vi "输入数据解析.vi"(0 "单个参数补充":dbl, 1 "从板号":dbl=1.0, 2 "主板二维码":string="BNET01", 3 "从板二维码":string="BNET01", 5 "主板引用":refnum<vi>, 7 "从板引用":refnum<vi>, 9 "主板选项":string="三级故障阀值", 11 "枚举":enum16{"主板", "从板"}(ring), 12 "快换":bool caption="快换写入") -> (4 "输出数组":dbl[][](array[numeric]), 6 "数组长度":dbl[](array[numeric]), 8 "循环次数":i32, 10 "命令":u32, 14 "名称":string[](array[string]), 15 "命令序号":u32[](array[numeric]))   [LabVIEW 2013] (continued)
                  frame Disabled {
                    n3517 = Unbundle By Name(w9112) -> ("温度过低"=w9111:dbl)
                    n3518 = call "输入分辨率计算-EV05.vi"("1字节?"=TRUE, "数值"=w9111, "偏移量"=-40.0, "分辨率"=1.0) -> ("高字节1"=w9114:dbl)  [unwired: 1 in, 6 out]
                  }
                  frame Enabled {
                  }
                }
                n3519 = Build Array(w9110) -> (w9109:i32[])
              }
              frame 4 {
                # "整组温度不均衡"
                n3520 = disable-structure shown="启用" {
                  disable-tunnel: [w9124 255 ("高字节1")] -> w9120
                  disable-tunnel: w9118 -> [w9122 _]
                  frame Disabled {
                    n3521 = Unbundle By Name(w9122) -> ("整组温度不均衡"=w9121:dbl)
                    n3522 = call "输入分辨率计算-EV05.vi"("1字节?"=TRUE, "数值"=w9121, "偏移量"=0.0, "分辨率"=1.0) -> ("高字节1"=w9124:dbl)  [unwired: 1 in, 6 out]
                  }
                  frame Enabled {
                  }
                }
                n3523 = Build Array(w9120) -> (w9119:i32[])
              }
              frame 5 {
                # "单组电压不均衡"
                n3524 = disable-structure shown="启用" {
                  disable-tunnel: [w9136 w9139] -> w9131
                  disable-tunnel: [w9134 w9139] -> w9129
                  disable-tunnel: w9128 -> [w9133 _]
                  frame Disabled {
                    n3525 = Unbundle By Name(w9133) -> ("单组电压不均衡"=w9132:dbl)
                    n3526 = call "输入分辨率计算-EV05.vi"("1字节?"=FALSE, "数值"=w9132, "偏移量"=0.0, "分辨率"=0.001) -> ("低字节"=w9134:dbl, "高字节1"=w9136:dbl)  [unwired: 1 in, 5 out]
                  }
                  frame Enabled {
                    w9139 = 255 ("高字节1")
                  }
                }
                n3527 = Build Array(w9131, w9129) -> (w9130:i32[])
              }
              frame 6 {
                # "整组电压不均衡"
                n3528 = disable-structure shown="启用" {
                  disable-tunnel: [w9148 w9151] -> w9143
                  disable-tunnel: [w9146 w9151] -> w9141
                  disable-tunnel: w9140 -> [w9145 _]
                  frame Disabled {
                    n3529 = Unbundle By Name(w9145) -> ("整组电压不均衡"=w9144:dbl)
                    n3530 = call "输入分辨率计算-EV05.vi"("1字节?"=FALSE, "数值"=w9144, "偏移量"=0.0, "分辨率"=0.001) -> ("低字节"=w9146:dbl, "高字节1"=w9148:dbl)  [unwired: 1 in, 5 out]
                  }
                  frame Enabled {
                    w9151 = 255 ("高字节1")
                  }
                }
                n3531 = Build Array(w9143, w9141) -> (w9142:i32[])
              }
              frame 7 {
                # "单体电压过高"
                n3532 = disable-structure shown="启用" {
                  disable-tunnel: [w9160 w9163] -> w9155
                  disable-tunnel: [w9158 w9163] -> w9153
                  disable-tunnel: w9152 -> [w9157 _]
                  frame Disabled {
                    n3533 = Unbundle By Name(w9157) -> ("单体电压过高"=w9156:dbl)
                    n3534 = call "输入分辨率计算-EV05.vi"("1字节?"=FALSE, "数值"=w9156, "偏移量"=0.0, "分辨率"=0.001) -> ("低字节"=w9158:dbl, "高字节1"=w9160:dbl)  [unwired: 1 in, 5 out]
                  }
                  frame Enabled {
                    w9163 = 255 ("高字节1")
                  }
                }
                n3535 = Build Array(w9155, w9153) -> (w9154:i32[])
              }
              frame 8 {
                # "单体电压过低"
                n3536 = disable-structure shown="启用" {
                  disable-tunnel: [w9172 w9175] -> w9167
                  disable-tunnel: [w9170 w9175] -> w9165
                  disable-tunnel: w9164 -> [w9169 _]
                  frame Disabled {
                    n3537 = Unbundle By Name(w9169) -> ("单体电压过低"=w9168:dbl)
                    n3538 = call "输入分辨率计算-EV05.vi"("1字节?"=FALSE, "数值"=w9168, "偏移量"=0.0, "分辨率"=0.001) -> ("低字节"=w9170:dbl, "高字节1"=w9172:dbl)  [unwired: 1 in, 5 out]
                  }
                  frame Enabled {
                    w9175 = 255 ("高字节1")
                  }
                }
                n3539 = Build Array(w9167, w9165) -> (w9166:i32[])
              }
              frame 9 {
                # "充电电流过高"
                n3540 = disable-structure shown="启用" {
                  disable-tunnel: [w9184 w9187] -> w9179
                  disable-tunnel: [w9182 w9187] -> w9177
                  disable-tunnel: w9176 -> [w9181 _]
                  frame Disabled {
                    n3541 = Unbundle By Name(w9181) -> ("充电电流过高"=w9180:dbl)
                    n3542 = call "输入分辨率计算-EV05.vi"("1字节?"=FALSE, "数值"=w9180, "偏移量"=-3000.0, "分辨率"=0.1) -> ("低字节"=w9182:dbl, "高字节1"=w9184:dbl)  [unwired: 1 in, 5 out]
                  }
                  frame Enabled {
                    w9187 = 255 ("高字节1")
                  }
                }
                n3543 = Build Array(w9179, w9177) -> (w9178:i32[])
              }
              frame 10 {
                # "放电电流过高"
                n3544 = disable-structure shown="启用" {
                  disable-tunnel: [w9196 w9199] -> w9191
                  disable-tunnel: [w9194 w9199] -> w9189
                  disable-tunnel: w9188 -> [w9193 _]
                  frame Disabled {
                    n3545 = Unbundle By Name(w9193) -> ("放电电流过高"=w9192:dbl)
                    n3546 = call "输入分辨率计算-EV05.vi"("1字节?"=FALSE, "数值"=w9192, "偏移量"=-3000.0, "分辨率"=0.1) -> ("低字节"=w9194:dbl, "高字节1"=w9196:dbl)  [unwired: 1 in, 5 out]
                  }
                  frame Enabled {
                    w9199 = 255 ("高字节1")
                  }
                }
                n3547 = Build Array(w9191, w9189) -> (w9190:i32[])
              }
              frame 11 {
                # "单组温度不均衡"
                n3548 = disable-structure shown="启用" {
                  disable-tunnel: [w9205 255 ("高字节1")] -> w9202
                  disable-tunnel: w9200 -> [w9204 _]
                  frame Enabled {
                    n3549 = Unbundle By Name(w9204) -> ("单组温度不均衡"=w9203:dbl)
                    n3550 = call "输入分辨率计算-EV05.vi"("1字节?"=TRUE, "数值"=w9203, "分辨率"=1.0) -> ("高字节1"=w9205:dbl)  [unwired: 2 in, 6 out]
                  }
                  frame Disabled {
                  }
                }
                n3551 = Build Array(w9202) -> (w9201:dbl[])
              }
              frame 12 {
                # "SOC过高"
                n3552 = Unbundle By Name(w9213) -> ("SOC过高"=w9212:dbl)
                n3553 = call "输入分辨率计算-EV05.vi"("1字节?"=FALSE, "数值"=w9212, "偏移量"=0.0, "分辨率"=0.1) -> ("低字节"=w9214:dbl, "高字节1"=w9215:dbl)  [unwired: 1 in, 5 out]
                n3554 = call "二进制解析-8.6.vi"("索引"=4, "数值"=w9215) -> ("低位子数组"=w9218:i32[])  [unwired: 3 out]
                n3555 = call "二进制解析-8.6.vi"("索引"=4, "数值"=w9214) -> ("低位子数组"=w9210:i32[], "高位子数组"=w9217:i32[])  [unwired: 2 out]
                n3556 = Insert Into Array(array=w9218, new element=w9217) -> (w9216:i32[])  [unwired: 1 in]
                n3557 = call "数值二进制转十进制-8.6.vi"("子数组"=w9216) -> ("十进制数值"=w9211:i32)  [unwired: 4 out]
                n3558 = disable-structure shown="启用" {
                  disable-tunnel: w9211 -> [w9226 _]
                  disable-tunnel: [w9226 255 ("高字节1")] -> w9209
                  disable-tunnel: w9210 -> [w9225 _]
                  disable-tunnel: [w9225 i32[] [] ("低位子数组 29")] -> _
                  frame Disabled {
                  }
                  frame Enabled {
                  }
                }
                n3559 = Build Array(w9209, w9209) -> (w9222:i32[])
              }
              frame 13 {
                # "SOC过低"
                n3560 = Unbundle By Name(w9234) -> ("SOC过低"=w9233:dbl)
                n3561 = call "输入分辨率计算-EV05.vi"("1字节?"=FALSE, "数值"=w9233, "偏移量"=0.0, "分辨率"=0.1) -> ("低字节"=w9231:dbl, "高字节1"=w9232:dbl)  [unwired: 1 in, 5 out]
                n3562 = call "二进制解析-8.6.vi"("索引"=4, "数值"=w9232) -> ("低位子数组"=w9230:i32[])  [unwired: 3 out]
                n3563 = disable-structure shown="启用" {
                  disable-tunnel: w9231 -> [w9241 _]
                  disable-tunnel: [w9241 255 ("高字节1")] -> w9229
                  disable-tunnel: w9230 -> [w9240 _]
                  disable-tunnel: [w9240 i32[] [] ("低位子数组")] -> _
                  frame Disabled {
                    (unwired) i32[] [] ("低位子数组 4")
                  }
                  frame Enabled {
                  }
                }
                n3564 = Build Array(w9229, w9229) -> (w9237:i32[])
              }
              frame 14 {
                # "内阻过大"
                n3565 = disable-structure shown="启用" {
                  disable-tunnel: w9246 -> [w9251 _]
                  disable-tunnel: [w9247 255 ("高字节1")] -> w9244
                  frame Disabled {
                    n3566 = Unbundle By Name(w9251) -> ("内阻过大"=w9250:dbl)
                    n3567 = call "输入分辨率计算-EV05.vi"("1字节?"=TRUE, "数值"=w9250, "分辨率"=0.1) -> ("高字节1"=w9247:dbl)  [unwired: 2 in, 6 out]
                  }
                  frame Enabled {
                  }
                }
                n3568 = Build Array(w9244) -> (w9245:i32[])
              }
              frame 15 {
                # "极柱温度过高"
                n3569 = disable-structure shown="启用" {
                  disable-tunnel: w9255 -> [w9261 _]
                  disable-tunnel: [w9257 255 ("高字节1")] -> w9253
                  frame Disabled {
                    n3570 = Unbundle By Name(w9261) -> ("极柱温度过高"=w9260:dbl)
                    n3571 = call "输入分辨率计算-EV05.vi"("1字节?"=TRUE, "数值"=w9260, "偏移量"=-40.0, "分辨率"=1.0) -> ("高字节1"=w9257:dbl)  [unwired: 1 in, 6 out]
                  }
                  frame Enabled {
                  }
                }
                n3572 = Build Array(w9253) -> (w9254:i32[])
              }
              frame 16 {
                # "SOH过低"
                n3573 = disable-structure shown="启用" {
                  disable-tunnel: [w9278 w9286] -> w9265
                  disable-tunnel: w9264 -> [w9275 _]
                  disable-tunnel: [w9267 w9286] -> w9263
                  frame Disabled {
                    n3574 = Unbundle By Name(w9275) -> ("SOH过低"=w9274:dbl)
                    n3575 = call "输入分辨率计算-EV05.vi"("1字节?"=FALSE, "数值"=w9274, "偏移量"=0.0, "分辨率"=0.1) -> ("低字节"=w9276:dbl, "高字节1"=w9277:dbl)  [unwired: 1 in, 5 out]
                    n3576 = call "二进制解析-8.6.vi"("索引"=4, "数值"=w9277) -> ("低位子数组"=w9280:i32[])  [unwired: 3 out]
                    n3577 = call "二进制解析-8.6.vi"("索引"=4, "数值"=w9276) -> ("低位子数组"=w9269:i32[], "高位子数组"=w9279:i32[])  [unwired: 2 out]
                    n3578 = call "二进制解析-8.6.vi"("索引"=4, "数值"=0) -> ("低位子数组"=w9270:i32[])  [unwired: 3 out]
                    n3579 = Insert Into Array(array=w9280, new element=w9279) -> (w9273:i32[])  [unwired: 1 in]
                    n3580 = Insert Into Array(array=w9269, new element=w9270) -> (w9268:i32[])  [unwired: 1 in]
                    n3581 = call "数值二进制转十进制-8.6.vi"("子数组"=w9273) -> ("十进制数值"=w9278:i32)  [unwired: 4 out]
                    n3582 = call "数值二进制转十进制-8.6.vi"("子数组"=w9268) -> ("十进制数值"=w9267:i32)  [unwired: 4 out]
                  }
                  frame Enabled {
                    w9286 = 255 ("高字节1")
                  }
                }
                n3583 = Build Array(w9265, w9263) -> (w9266:i32[])
              }
            }
            n3584 = Insert Into Array(array=w9072, new element=w9073) -> (w9071:dbl[])  [unwired: 1 in]
          }
          n3585 = Build Array(w9068) -> (w9067:dbl[][])
          n3586 = Build Array("三级故障阀值") -> (w9058:string[])
        }
        frame "内阻过大" {
          n3587 = Unbundle By Name(w9292) -> ("一级故障"=w9293:refnum<vi>)
          n3588 = property class="Clust (严格)"(reference=w9293) -> ("Value"=w9291:T4)  [unwired: 1 in, 2 out]
          n3589 = for {
            N: 17 -> [_]
            tunnel: w9291 -> [w9303]
            shift-right: [w9300] -> w9297
            shift-left: dbl[] [] -> [w9301]
            i -> [w9304]
            n3590 = case shown="13" w9304 {
              tunnel: w9303 -> [w9305 w9316 w9327 w9337 w9347 w9357 w9369 w9381 w9393 w9405 w9417 w9429 w9443 w9464 w9476 w9485 w9494]
              tunnel: [w9306 w9317 w9328 w9338 w9348 w9359 w9371 w9383 w9395 w9407 w9419 w9430 w9452 w9467 w9475 w9484 w9496] -> w9302
              frame 0, Default {
                # "总电压过高"
                n3591 = disable-structure shown="启用" {
                  disable-tunnel: [w9312 w9315] -> w9308
                  disable-tunnel: [w9311 w9315] -> w9307
                  disable-tunnel: w9305 -> [w9310 _]
                  frame Disabled {
                    n3592 = Unbundle By Name(w9310) -> ("总电压过高"=w9309:dbl)
                    n3593 = call "输入分辨率计算-EV05.vi"("1字节?"=FALSE, "数值"=w9309, "分辨率"=0.1) -> ("低字节"=w9312:dbl, "高字节1"=w9311:dbl)  [unwired: 2 in, 5 out]
                  }
                  frame Enabled {
                    w9315 = 255 ("高字节1")
                  }
                }
                n3594 = Build Array(w9307, w9308) -> (w9306:i32[])
              }
              frame 1 {
                # "总电压过低"
                n3595 = disable-structure shown="启用" {
                  disable-tunnel: [w9323 w9326] -> w9319
                  disable-tunnel: [w9322 w9326] -> w9318
                  disable-tunnel: w9316 -> [w9321 _]
                  frame Disabled {
                    n3596 = Unbundle By Name(w9321) -> ("总电压过低"=w9320:dbl)
                    n3597 = call "输入分辨率计算-EV05.vi"("1字节?"=FALSE, "数值"=w9320, "分辨率"=0.1) -> ("低字节"=w9323:dbl, "高字节1"=w9322:dbl)  [unwired: 2 in, 5 out]
                  }
                  frame Enabled {
                    w9326 = 255 ("高字节1")
                  }
                }
                n3598 = Build Array(w9318, w9319) -> (w9317:i32[])
              }
              frame 2 {
                # "温度过高"
                n3599 = disable-structure shown="启用" {
                  disable-tunnel: [w9333 255 ("高字节1")] -> w9329
                  disable-tunnel: w9327 -> [w9331 _]
                  frame Disabled {
                    n3600 = Unbundle By Name(w9331) -> ("温度过高"=w9330:dbl)
                    n3601 = call "输入分辨率计算-EV05.vi"("1字节?"=TRUE, "数值"=w9330, "偏移量"=-40.0, "分辨率"=1.0) -> ("高字节1"=w9333:dbl)  [unwired: 1 in, 6 out]
                  }
                  frame Enabled {
                  }
                }
                n3602 = Build Array(w9329) -> (w9328:i32[])
              }
              frame 3 {
                # "温度过低"
                n3603 = disable-structure shown="启用" {
                  disable-tunnel: [w9343 255 ("高字节1")] -> w9339
                  disable-tunnel: w9337 -> [w9341 _]
                  frame Disabled {
                    n3604 = Unbundle By Name(w9341) -> ("温度过低"=w9340:dbl)
                    n3605 = call "输入分辨率计算-EV05.vi"("1字节?"=TRUE, "数值"=w9340, "偏移量"=-40.0, "分辨率"=1.0) -> ("高字节1"=w9343:dbl)  [unwired: 1 in, 6 out]
                  }
                  frame Enabled {
                  }
                }
                n3606 = Build Array(w9339) -> (w9338:i32[])
              }
              frame 4 {
                # "整组温度不均衡"
                n3607 = disable-structure shown="启用" {
                  disable-tunnel: [w9353 255 ("高字节1")] -> w9349
                  disable-tunnel: w9347 -> [w9351 _]
                  frame Disabled {
                    n3608 = Unbundle By Name(w9351) -> ("整组温度不均衡"=w9350:dbl)
                    n3609 = call "输入分辨率计算-EV05.vi"("1字节?"=TRUE, "数值"=w9350, "偏移量"=0.0, "分辨率"=1.0) -> ("高字节1"=w9353:dbl)  [unwired: 1 in, 6 out]
                  }
                  frame Enabled {
                  }
                }
                n3610 = Build Array(w9349) -> (w9348:i32[])
              }
              frame 5 {
                # "单组电压不均衡"
                n3611 = disable-structure shown="启用" {
                  disable-tunnel: [w9365 w9368] -> w9360
                  disable-tunnel: [w9363 w9368] -> w9358
                  disable-tunnel: w9357 -> [w9362 _]
                  frame Disabled {
                    n3612 = Unbundle By Name(w9362) -> ("单组电压不均衡"=w9361:dbl)
                    n3613 = call "输入分辨率计算-EV05.vi"("1字节?"=FALSE, "数值"=w9361, "偏移量"=0.0, "分辨率"=0.001) -> ("低字节"=w9363:dbl, "高字节1"=w9365:dbl)  [unwired: 1 in, 5 out]
                  }
                  frame Enabled {
                    w9368 = 255 ("高字节1")
                  }
                }
                n3614 = Build Array(w9360, w9358) -> (w9359:i32[])
              }
              frame 6 {
                # "整组电压不均衡"
                n3615 = disable-structure shown="启用" {
                  disable-tunnel: [w9377 w9380] -> w9372
                  disable-tunnel: [w9375 w9380] -> w9370
                  disable-tunnel: w9369 -> [w9374 _]
                  frame Disabled {
                    n3616 = Unbundle By Name(w9374) -> ("整组电压不均衡"=w9373:dbl)
                    n3617 = call "输入分辨率计算-EV05.vi"("1字节?"=FALSE, "数值"=w9373, "偏移量"=0.0, "分辨率"=0.001) -> ("低字节"=w9375:dbl, "高字节1"=w9377:dbl)  [unwired: 1 in, 5 out]
                  }
                  frame Enabled {
                    w9380 = 255 ("高字节1")
                  }
                }
                n3618 = Build Array(w9372, w9370) -> (w9371:i32[])
              }
              frame 7 {
                # "单体电压过高"
                n3619 = disable-structure shown="启用" {
                  disable-tunnel: [w9389 w9392] -> w9384
                  disable-tunnel: [w9387 w9392] -> w9382
                  disable-tunnel: w9381 -> [w9386 _]
                  frame Disabled {
                    n3620 = Unbundle By Name(w9386) -> ("单体电压过高"=w9385:dbl)
                    n3621 = call "输入分辨率计算-EV05.vi"("1字节?"=FALSE, "数值"=w9385, "偏移量"=0.0, "分辨率"=0.001) -> ("低字节"=w9387:dbl, "高字节1"=w9389:dbl)  [unwired: 1 in, 5 out]
                  }
                  frame Enabled {
                    w9392 = 255 ("高字节1")
                  }
                }
                n3622 = Build Array(w9384, w9382) -> (w9383:i32[])
              }
              frame 8 {
                # "单体电压过低"
                n3623 = disable-structure shown="启用" {
                  disable-tunnel: [w9401 w9404] -> w9396
                  disable-tunnel: [w9399 w9404] -> w9394
                  disable-tunnel: w9393 -> [w9398 _]
                  frame Disabled {
                    n3624 = Unbundle By Name(w9398) -> ("单体电压过低"=w9397:dbl)
                    n3625 = call "输入分辨率计算-EV05.vi"("1字节?"=FALSE, "数值"=w9397, "偏移量"=0.0, "分辨率"=0.001) -> ("低字节"=w9399:dbl, "高字节1"=w9401:dbl)  [unwired: 1 in, 5 out]
                  }
                  frame Enabled {
                    w9404 = 255 ("高字节1")
                  }
                }
                n3626 = Build Array(w9396, w9394) -> (w9395:i32[])
              }
              frame 9 {
                # "充电电流过高"
                n3627 = disable-structure shown="启用" {
                  disable-tunnel: [w9413 w9416] -> w9408
                  disable-tunnel: [w9411 w9416] -> w9406
                  disable-tunnel: w9405 -> [w9410 _]
                  frame Disabled {
                    n3628 = Unbundle By Name(w9410) -> ("充电电流过高"=w9409:dbl)
                    n3629 = call "输入分辨率计算-EV05.vi"("1字节?"=FALSE, "数值"=w9409, "偏移量"=-3000.0, "分辨率"=0.1) -> ("低字节"=w9411:dbl, "高字节1"=w9413:dbl)  [unwired: 1 in, 5 out]
                  }
                  frame Enabled {
                    w9416 = 255 ("高字节1")
                  }
                }
                n3630 = Build Array(w9408, w9406) -> (w9407:i32[])
              }
              frame 10 {
                # "放电电流过高"
                n3631 = disable-structure shown="启用" {
                  disable-tunnel: [w9425 w9428] -> w9420
                  disable-tunnel: [w9423 w9428] -> w9418
                  disable-tunnel: w9417 -> [w9422 _]
                  frame Disabled {
                    n3632 = Unbundle By Name(w9422) -> ("放电电流过高"=w9421:dbl)
                    n3633 = call "输入分辨率计算-EV05.vi"("1字节?"=FALSE, "数值"=w9421, "偏移量"=-3000.0, "分辨率"=0.1) -> ("低字节"=w9423:dbl, "高字节1"=w9425:dbl)  [unwired: 1 in, 5 out]
                  }
                  frame Enabled {
                    w9428 = 255 ("高字节1")
                  }
                }
                n3634 = Build Array(w9420, w9418) -> (w9419:i32[])
              }
              frame 11 {
                # "单组温度不均衡"
                n3635 = disable-structure shown="启用" {
                  disable-tunnel: [w9435 255 ("高字节1")] -> w9431
                  disable-tunnel: w9429 -> [w9433 _]
                  frame Disabled {
                    n3636 = Unbundle By Name(w9433) -> ("单组温度不均衡"=w9432:dbl)
                    n3637 = call "输入分辨率计算-EV05.vi"("1字节?"=TRUE, "数值"=w9432, "偏移量"=0.0, "分辨率"=1.0) -> ("高字节1"=w9435:dbl)  [unwired: 1 in, 6 out]
                  }
                  frame Enabled {
                  }
                }
                n3638 = Build Array(w9431) -> (w9430:i32[])
              }
              frame 12 {
                # "SOC过高"
                n3639 = Unbundle By Name(w9443) -> ("SOC过高"=w9442:dbl)
                n3640 = call "输入分辨率计算-EV05.vi"("1字节?"=FALSE, "数值"=w9442, "偏移量"=0.0, "分辨率"=0.1) -> ("低字节"=w9444:dbl, "高字节1"=w9445:dbl)  [unwired: 1 in, 5 out]
                n3641 = call "二进制解析-8.6.vi"("索引"=4, "数值"=w9445) -> ("低位子数组"=w9448:i32[])  [unwired: 3 out]
                n3642 = call "二进制解析-8.6.vi"("索引"=4, "数值"=w9444) -> ("低位子数组"=w9440:i32[], "高位子数组"=w9447:i32[])  [unwired: 2 out]
                n3643 = Insert Into Array(array=w9448, new element=w9447) -> (w9446:i32[])  [unwired: 1 in]
                n3644 = call "数值二进制转十进制-8.6.vi"("子数组"=w9446) -> ("十进制数值"=w9441:i32)  [unwired: 4 out]
                n3645 = disable-structure shown="启用" {
                  disable-tunnel: w9441 -> [w9456 _]
                  disable-tunnel: [w9456 255 ("高字节1")] -> w9439
                  disable-tunnel: w9440 -> [w9455 _]
                  disable-tunnel: [w9455 i32[] [] ("低位子数组 29")] -> _
                  frame Disabled {
                  }
                  frame Enabled {
                  }
                }
                n3646 = Build Array(w9439, w9439) -> (w9452:i32[])
              }
              frame 13 {
                # "SOC过低"
                n3647 = Unbundle By Name(w9464) -> ("SOC过低"=w9463:dbl)
                n3648 = call "输入分辨率计算-EV05.vi"("1字节?"=FALSE, "数值"=w9463, "偏移量"=0.0, "分辨率"=0.1) -> ("低字节"=w9461:dbl, "高字节1"=w9462:dbl)  [unwired: 1 in, 5 out]
                n3649 = call "二进制解析-8.6.vi"("索引"=4, "数值"=w9462) -> ("低位子数组"=w9460:i32[])  [unwired: 3 out]
                n3650 = disable-structure shown="启用" {
                  disable-tunnel: w9461 -> [w9471 _]
                  disable-tunnel: [w9471 255 ("高字节1")] -> w9459
                  disable-tunnel: w9460 -> [w9470 _]
                  disable-tunnel: [w9470 i32[] [] ("低位子数组")] -> _
                  frame Disabled {
                    (unwired) i32[] [] ("低位子数组 4")
                  }
                  frame Enabled {
                  }
                }
                n3651 = Build Array(w9459, w9459) -> (w9467:i32[])
              }
              frame 14 {
                # "内阻过大"
                n3652 = disable-structure shown="启用" {
                  disable-tunnel: w9476 -> [w9481 _]
                  disable-tunnel: [w9477 255 ("高字节1")] -> w9474
                  frame Enabled {
                    n3653 = Unbundle By Name(w9481) -> ("内阻过大"=w9480:dbl)
                    n3654 = call "输入分辨率计算-EV05.vi"("1字节?"=TRUE, "数值"=w9480, "分辨率"=0.1) -> ("高字节1"=w9477:dbl)  [unwired: 2 in, 6 out]
                  }
                  frame Disabled {
                  }
                }
                n3655 = Build Array(w9474) -> (w9475:dbl[])
              }
              frame 15 {
                # "极柱温度过高"
                n3656 = disable-structure shown="启用" {
                  disable-tunnel: w9485 -> [w9491 _]
                  disable-tunnel: [w9487 255 ("高字节1")] -> w9483
                  frame Disabled {
                    n3657 = Unbundle By Name(w9491) -> ("极柱温度过高"=w9490:dbl)
                    n3658 = call "输入分辨率计算-EV05.vi"("1字节?"=TRUE, "数值"=w9490, "偏移量"=-40.0, "分辨率"=1.0) -> ("高字节1"=w9487:dbl)  [unwired: 1 in, 6 out]
                  }
                  frame Enabled {
                  }
                }
                n3659 = Build Array(w9483) -> (w9484:i32[])
              }
              frame 16 {
                # "SOH过低"
                n3660 = disable-structure shown="启用" {
                  disable-tunnel: [w9508 w9516] -> w9495
                  disable-tunnel: w9494 -> [w9505 _]
                  disable-tunnel: [w9497 w9516] -> w9493
                  frame Disabled {
                    n3661 = Unbundle By Name(w9505) -> ("SOH过低"=w9504:dbl)
                    n3662 = call "输入分辨率计算-EV05.vi"("1字节?"=FALSE, "数值"=w9504, "偏移量"=0.0, "分辨率"=0.1) -> ("低字节"=w9506:dbl, "高字节1"=w9507:dbl)  [unwired: 1 in, 5 out]
                    n3663 = call "二进制解析-8.6.vi"("索引"=4, "数值"=w9507) -> ("低位子数组"=w9510:i32[])  [unwired: 3 out]
                    n3664 = call "二进制解析-8.6.vi"("索引"=4, "数值"=w9506) -> ("低位子数组"=w9499:i32[], "高位子数组"=w9509:i32[])  [unwired: 2 out]
                    n3665 = call "二进制解析-8.6.vi"("索引"=4, "数值"=0) -> ("低位子数组"=w9500:i32[])  [unwired: 3 out]
                    n3666 = Insert Into Array(array=w9510, new element=w9509) -> (w9503:i32[])  [unwired: 1 in]
                    n3667 = Insert Into Array(array=w9499, new element=w9500) -> (w9498:i32[])  [unwired: 1 in]
                    n3668 = call "数值二进制转十进制-8.6.vi"("子数组"=w9503) -> ("十进制数值"=w9508:i32)  [unwired: 4 out]
                    n3669 = call "数值二进制转十进制-8.6.vi"("子数组"=w9498) -> ("十进制数值"=w9497:i32)  [unwired: 4 out]
                  }
                  frame Enabled {
                    w9516 = 255 ("高字节1")
                  }
                }
                n3670 = Build Array(w9495, w9493) -> (w9496:i32[])
              }
            }
            n3671 = Insert Into Array(array=w9301, new element=w9302) -> (w9300:dbl[])  [unwired: 1 in]
          }
          n3672 = Build Array(w9297) -> (w9296:dbl[][])
          n3673 = Build Array("一级故障阀值") -> (w9287:string[])
        }
        frame "内阻过大(2)" {
          n3674 = Unbundle By Name(w9522) -> ("一级故障 2"=w9523:refnum<vi>)
          n3675 = property class="Clust (严格)"(reference=w9523) -> ("Value"=w9521:T4)  [unwired: 1 in, 2 out]
          n3676 = for {
            N: 17 -> [_]
            tunnel: w9521 -> [w9533]
            shift-right: [w9530] -> w9527
            shift-left: dbl[] [] -> [w9531]
            i -> [w9534]
            n3677 = case shown="13" w9534 {
              tunnel: w9533 -> [w9535 w9546 w9557 w9567 w9577 w9587 w9599 w9611 w9623 w9635 w9647 w9659 w9673 w9694 w9706 w9715 w9724]
              tunnel: [w9536 w9547 w9558 w9568 w9578 w9589 w9601 w9613 w9625 w9637 w9649 w9660 w9682 w9697 w9705 w9714 w9726] -> w9532
              frame 0, Default {
                # "总电压过高"
                n3678 = disable-structure shown="启用" {
                  disable-tunnel: [w9542 w9545] -> w9538
                  disable-tunnel: [w9541 w9545] -> w9537
                  disable-tunnel: w9535 -> [w9540 _]
                  frame Disabled {
                    n3679 = Unbundle By Name(w9540) -> ("总电压过高"=w9539:dbl)
                    n3680 = call "输入分辨率计算-EV05.vi"("1字节?"=FALSE, "数值"=w9539, "分辨率"=0.1) -> ("低字节"=w9542:dbl, "高字节1"=w9541:dbl)  [unwired: 2 in, 5 out]
                  }
                  frame Enabled {
                    w9545 = 255 ("高字节1")
                  }
                }
                n3681 = Build Array(w9537, w9538) -> (w9536:i32[])
              }
              frame 1 {
                # "总电压过低"
                n3682 = disable-structure shown="启用" {
                  disable-tunnel: [w9553 w9556] -> w9549
                  disable-tunnel: [w9552 w9556] -> w9548
                  disable-tunnel: w9546 -> [w9551 _]
                  frame Disabled {
                    n3683 = Unbundle By Name(w9551) -> ("总电压过低"=w9550:dbl)
                    n3684 = call "输入分辨率计算-EV05.vi"("1字节?"=FALSE, "数值"=w9550, "分辨率"=0.1) -> ("低字节"=w9553:dbl, "高字节1"=w9552:dbl)  [unwired: 2 in, 5 out]
                  }
                  frame Enabled {
                    w9556 = 255 ("高字节1")
                  }
                }
                n3685 = Build Array(w9548, w9549) -> (w9547:i32[])
              }
              frame 2 {
                # "温度过高"
                n3686 = disable-structure shown="启用" {
                  disable-tunnel: [w9563 255 ("高字节1")] -> w9559
                  disable-tunnel: w9557 -> [w9561 _]
                  frame Disabled {
                    n3687 = Unbundle By Name(w9561) -> ("温度过高"=w9560:dbl)
                    n3688 = call "输入分辨率计算-EV05.vi"("1字节?"=TRUE, "数值"=w9560, "偏移量"=-40.0, "分辨率"=1.0) -> ("高字节1"=w9563:dbl)  [unwired: 1 in, 6 out]
                  }
                  frame Enabled {
                  }
                }
                n3689 = Build Array(w9559) -> (w9558:i32[])
              }
              frame 3 {
                # "温度过低"
                n3690 = disable-structure shown="启用" {
                  disable-tunnel: [w9573 255 ("高字节1")] -> w9569
                  disable-tunnel: w9567 -> [w9571 _]
                  frame Disabled {
                    n3691 = Unbundle By Name(w9571) -> ("温度过低"=w9570:dbl)
                    n3692 = call "输入分辨率计算-EV05.vi"("1字节?"=TRUE, "数值"=w9570, "偏移量"=-40.0, "分辨率"=1.0) -> ("高字节1"=w9573:dbl)  [unwired: 1 in, 6 out]
                  }
                  frame Enabled {
                  }
                }
                n3693 = Build Array(w9569) -> (w9568:i32[])
              }
              frame 4 {
                # "整组温度不均衡"
                n3694 = disable-structure shown="启用" {
                  disable-tunnel: [w9583 255 ("高字节1")] -> w9579
                  disable-tunnel: w9577 -> [w9581 _]
                  frame Disabled {
                    n3695 = Unbundle By Name(w9581) -> ("整组温度不均衡"=w9580:dbl)
                    n3696 = call "输入分辨率计算-EV05.vi"("1字节?"=TRUE, "数值"=w9580, "偏移量"=0.0, "分辨率"=1.0) -> ("高字节1"=w9583:dbl)  [unwired: 1 in, 6 out]
                  }
                  frame Enabled {
                  }
                }
                n3697 = Build Array(w9579) -> (w9578:i32[])
              }
              frame 5 {
                # "单组电压不均衡"
                n3698 = disable-structure shown="启用" {
                  disable-tunnel: [w9595 w9598] -> w9590
                  disable-tunnel: [w9593 w9598] -> w9588
                  disable-tunnel: w9587 -> [w9592 _]
                  frame Disabled {
                    n3699 = Unbundle By Name(w9592) -> ("单组电压不均衡"=w9591:dbl)
                    n3700 = call "输入分辨率计算-EV05.vi"("1字节?"=FALSE, "数值"=w9591, "偏移量"=0.0, "分辨率"=0.001) -> ("低字节"=w9593:dbl, "高字节1"=w9595:dbl)  [unwired: 1 in, 5 out]
                  }
                  frame Enabled {
                    w9598 = 255 ("高字节1")
                  }
                }
                n3701 = Build Array(w9590, w9588) -> (w9589:i32[])
              }
              frame 6 {
                # "整组电压不均衡"
                n3702 = disable-structure shown="启用" {
                  disable-tunnel: [w9607 w9610] -> w9602
                  disable-tunnel: [w9605 w9610] -> w9600
                  disable-tunnel: w9599 -> [w9604 _]
                  frame Disabled {
                    n3703 = Unbundle By Name(w9604) -> ("整组电压不均衡"=w9603:dbl)
                    n3704 = call "输入分辨率计算-EV05.vi"("1字节?"=FALSE, "数值"=w9603, "偏移量"=0.0, "分辨率"=0.001) -> ("低字节"=w9605:dbl, "高字节1"=w9607:dbl)  [unwired: 1 in, 5 out]
                  }
                  frame Enabled {
                    w9610 = 255 ("高字节1")
                  }
                }
                n3705 = Build Array(w9602, w9600) -> (w9601:i32[])
              }
              frame 7 {
                # "单体电压过高"
                n3706 = disable-structure shown="启用" {
                  disable-tunnel: [w9619 w9622] -> w9614
                  disable-tunnel: [w9617 w9622] -> w9612
                  disable-tunnel: w9611 -> [w9616 _]
                  frame Disabled {
                    n3707 = Unbundle By Name(w9616) -> ("单体电压过高"=w9615:dbl)
                    n3708 = call "输入分辨率计算-EV05.vi"("1字节?"=FALSE, "数值"=w9615, "偏移量"=0.0, "分辨率"=0.001) -> ("低字节"=w9617:dbl, "高字节1"=w9619:dbl)  [unwired: 1 in, 5 out]
                  }
                  frame Enabled {
                    w9622 = 255 ("高字节1")
                  }
                }
                n3709 = Build Array(w9614, w9612) -> (w9613:i32[])
              }
              frame 8 {
                # "单体电压过低"
                n3710 = disable-structure shown="启用" {
                  disable-tunnel: [w9631 w9634] -> w9626
                  disable-tunnel: [w9629 w9634] -> w9624
                  disable-tunnel: w9623 -> [w9628 _]
                  frame Disabled {
                    n3711 = Unbundle By Name(w9628) -> ("单体电压过低"=w9627:dbl)
                    n3712 = call "输入分辨率计算-EV05.vi"("1字节?"=FALSE, "数值"=w9627, "偏移量"=0.0, "分辨率"=0.001) -> ("低字节"=w9629:dbl, "高字节1"=w9631:dbl)  [unwired: 1 in, 5 out]
                  }
                  frame Enabled {
                    w9634 = 255 ("高字节1")
                  }
                }
                n3713 = Build Array(w9626, w9624) -> (w9625:i32[])
              }
              frame 9 {
                # "充电电流过高"
                n3714 = disable-structure shown="启用" {
                  disable-tunnel: [w9643 w9646] -> w9638
                  disable-tunnel: [w9641 w9646] -> w9636
                  disable-tunnel: w9635 -> [w9640 _]
                  frame Disabled {
                    n3715 = Unbundle By Name(w9640) -> ("充电电流过高"=w9639:dbl)
                    n3716 = call "输入分辨率计算-EV05.vi"("1字节?"=FALSE, "数值"=w9639, "偏移量"=-3000.0, "分辨率"=0.1) -> ("低字节"=w9641:dbl, "高字节1"=w9643:dbl)  [unwired: 1 in, 5 out]
                  }
                  frame Enabled {
                    w9646 = 255 ("高字节1")
                  }
                }
                n3717 = Build Array(w9638, w9636) -> (w9637:i32[])
              }
              frame 10 {
                # "放电电流过高"
                n3718 = disable-structure shown="启用" {
                  disable-tunnel: [w9655 w9658] -> w9650
                  disable-tunnel: [w9653 w9658] -> w9648
                  disable-tunnel: w9647 -> [w9652 _]
                  frame Disabled {
                    n3719 = Unbundle By Name(w9652) -> ("放电电流过高"=w9651:dbl)
                    n3720 = call "输入分辨率计算-EV05.vi"("1字节?"=FALSE, "数值"=w9651, "偏移量"=-3000.0, "分辨率"=0.1) -> ("低字节"=w9653:dbl, "高字节1"=w9655:dbl)  [unwired: 1 in, 5 out]
                  }
                  frame Enabled {
                    w9658 = 255 ("高字节1")
                  }
                }
                n3721 = Build Array(w9650, w9648) -> (w9649:i32[])
              }
              frame 11 {
                # "单组温度不均衡"
                n3722 = disable-structure shown="启用" {
                  disable-tunnel: [w9665 255 ("高字节1")] -> w9661
                  disable-tunnel: w9659 -> [w9663 _]
                  frame Disabled {
                    n3723 = Unbundle By Name(w9663) -> ("单组温度不均衡"=w9662:dbl)
                    n3724 = call "输入分辨率计算-EV05.vi"("1字节?"=TRUE, "数值"=w9662, "偏移量"=0.0, "分辨率"=1.0) -> ("高字节1"=w9665:dbl)  [unwired: 1 in, 6 out]
                  }
                  frame Enabled {
                  }
                }
                n3725 = Build Array(w9661) -> (w9660:i32[])
              }
              frame 12 {
                # "SOC过高"
                n3726 = Unbundle By Name(w9673) -> ("SOC过高"=w9672:dbl)
                n3727 = call "输入分辨率计算-EV05.vi"("1字节?"=FALSE, "数值"=w9672, "偏移量"=0.0, "分辨率"=0.1) -> ("低字节"=w9674:dbl, "高字节1"=w9675:dbl)  [unwired: 1 in, 5 out]
                n3728 = call "二进制解析-8.6.vi"("索引"=4, "数值"=w9675) -> ("低位子数组"=w9678:i32[])  [unwired: 3 out]
                n3729 = call "二进制解析-8.6.vi"("索引"=4, "数值"=w9674) -> ("低位子数组"=w9670:i32[], "高位子数组"=w9677:i32[])  [unwired: 2 out]
                n3730 = Insert Into Array(array=w9678, new element=w9677) -> (w9676:i32[])  [unwired: 1 in]
                n3731 = call "数值二进制转十进制-8.6.vi"("子数组"=w9676) -> ("十进制数值"=w9671:i32)  [unwired: 4 out]
                n3732 = disable-structure shown="启用" {
                  disable-tunnel: w9671 -> [w9686 _]
                  disable-tunnel: [w9686 255 ("高字节1")] -> w9669
                  disable-tunnel: w9670 -> [w9685 _]
                  disable-tunnel: [w9685 i32[] [] ("低位子数组 29")] -> _
                  frame Disabled {
                  }
                  frame Enabled {
                  }
                }
                n3733 = Build Array(w9669, w9669) -> (w9682:i32[])
              }
              frame 13 {
                # "SOC过低"
                n3734 = Unbundle By Name(w9694) -> ("SOC过低"=w9693:dbl)
                n3735 = call "输入分辨率计算-EV05.vi"("1字节?"=FALSE, "数值"=w9693, "偏移量"=0.0, "分辨率"=0.1) -> ("低字节"=w9691:dbl, "高字节1"=w9692:dbl)  [unwired: 1 in, 5 out]
                n3736 = call "二进制解析-8.6.vi"("索引"=4, "数值"=w9692) -> ("低位子数组"=w9690:i32[])  [unwired: 3 out]
                n3737 = disable-structure shown="启用" {
                  disable-tunnel: w9691 -> [w9701 _]
                  disable-tunnel: [w9701 255 ("高字节1")] -> w9689
                  disable-tunnel: w9690 -> [w9700 _]
                  disable-tunnel: [w9700 i32[] [] ("低位子数组")] -> _
                  frame Disabled {
                    (unwired) i32[] [] ("低位子数组 4")
                  }
                  frame Enabled {
                  }
                }
                n3738 = Build Array(w9689, w9689) -> (w9697:i32[])
              }
              frame 14 {
                # "内阻过大"
                n3739 = disable-structure shown="启用" {
                  disable-tunnel: w9706 -> [w9711 _]
                  disable-tunnel: [w9707 255 ("高字节1")] -> w9704
                  frame Enabled {
                    n3740 = Unbundle By Name(w9711) -> ("内阻过大"=w9710:dbl)
                    n3741 = call "输入分辨率计算-EV05.vi"("1字节?"=TRUE, "数值"=w9710, "分辨率"=0.1) -> ("高字节1"=w9707:dbl)  [unwired: 2 in, 6 out]
                  }
                  frame Disabled {
                  }
                }
                n3742 = Build Array(w9704) -> (w9705:dbl[])
              }
              frame 15 {
                # "极柱温度过高"
                n3743 = disable-structure shown="启用" {
                  disable-tunnel: w9715 -> [w9721 _]
                  disable-tunnel: [w9717 255 ("高字节1")] -> w9713
                  frame Disabled {
                    n3744 = Unbundle By Name(w9721) -> ("极柱温度过高"=w9720:dbl)
                    n3745 = call "输入分辨率计算-EV05.vi"("1字节?"=TRUE, "数值"=w9720, "偏移量"=-40.0, "分辨率"=1.0) -> ("高字节1"=w9717:dbl)  [unwired: 1 in, 6 out]
                  }
                  frame Enabled {
                  }
                }
                n3746 = Build Array(w9713) -> (w9714:i32[])
              }
              frame 16 {
                # "SOH过低"
                n3747 = disable-structure shown="启用" {
                  disable-tunnel: [w9738 w9746] -> w9725
                  disable-tunnel: w9724 -> [w9735 _]
                  disable-tunnel: [w9727 w9746] -> w9723
                  frame Disabled {
                    n3748 = Unbundle By Name(w9735) -> ("SOH过低"=w9734:dbl)
                    n3749 = call "输入分辨率计算-EV05.vi"("1字节?"=FALSE, "数值"=w9734, "偏移量"=0.0, "分辨率"=0.1) -> ("低字节"=w9736:dbl, "高字节1"=w9737:dbl)  [unwired: 1 in, 5 out]
                    n3750 = call "二进制解析-8.6.vi"("索引"=4, "数值"=w9737) -> ("低位子数组"=w9740:i32[])  [unwired: 3 out]
                    n3751 = call "二进制解析-8.6.vi"("索引"=4, "数值"=w9736) -> ("低位子数组"=w9729:i32[], "高位子数组"=w9739:i32[])  [unwired: 2 out]
                    n3752 = call "二进制解析-8.6.vi"("索引"=4, "数值"=0) -> ("低位子数组"=w9730:i32[])  [unwired: 3 out]
                    n3753 = Insert Into Array(array=w9740, new element=w9739) -> (w9733:i32[])  [unwired: 1 in]
                    n3754 = Insert Into Array(array=w9729, new element=w9730) -> (w9728:i32[])  [unwired: 1 in]
                    n3755 = call "数值二进制转十进制-8.6.vi"("子数组"=w9733) -> ("十进制数值"=w9738:i32)  [unwired: 4 out]
                    n3756 = call "数值二进制转十进制-8.6.vi"("子数组"=w9728) -> ("十进制数值"=w9727:i32)  [unwired: 4 out]
                  }
                  frame Enabled {
                    w9746 = 255 ("高字节1")
                  }
                }
                n3757 = Build Array(w9725, w9723) -> (w9726:i32[])
              }
            }
            n3758 = Insert Into Array(array=w9531, new element=w9532) -> (w9530:dbl[])  [unwired: 1 in]
          }
          n3759 = Build Array(w9527) -> (w9526:dbl[][])
          n3760 = Build Array("二级故障阀值") -> (w9517:string[])
        }
        frame "内阻过大(3)" {
          n3761 = Unbundle By Name(w9752) -> ("一级故障 3"=w9753:refnum<vi>)
          n3762 = property class="Clust (严格)"(reference=w9753) -> ("Value"=w9751:T4)  [unwired: 1 in, 2 out]
          n3763 = for {
            N: 17 -> [_]
            tunnel: w9751 -> [w9763]
            shift-right: [w9760] -> w9757
            shift-left: dbl[] [] -> [w9761]
            i -> [w9764]
            n3764 = case shown="13" w9764 {
              tunnel: w9763 -> [w9765 w9776 w9787 w9797 w9807 w9817 w9829 w9841 w9853 w9865 w9877 w9889 w9903 w9924 w9936 w9945 w9954]
              tunnel: [w9766 w9777 w9788 w9798 w9808 w9819 w9831 w9843 w9855 w9867 w9879 w9890 w9912 w9927 w9935 w9944 w9956] -> w9762
              frame 0, Default {
                # "总电压过高"
                n3765 = disable-structure shown="启用" {
                  disable-tunnel: [w9772 w9775] -> w9768
                  disable-tunnel: [w9771 w9775] -> w9767
                  disable-tunnel: w9765 -> [w9770 _]
                  frame Disabled {
                    n3766 = Unbundle By Name(w9770) -> ("总电压过高"=w9769:dbl)
                    n3767 = call "输入分辨率计算-EV05.vi"("1字节?"=FALSE, "数值"=w9769, "分辨率"=0.1) -> ("低字节"=w9772:dbl, "高字节1"=w9771:dbl)  [unwired: 2 in, 5 out]
                  }
                  frame Enabled {
                    w9775 = 255 ("高字节1")
                  }
                }
                n3768 = Build Array(w9767, w9768) -> (w9766:i32[])
              }
              frame 1 {
                # "总电压过低"
                n3769 = disable-structure shown="启用" {
                  disable-tunnel: [w9783 w9786] -> w9779
                  disable-tunnel: [w9782 w9786] -> w9778
                  disable-tunnel: w9776 -> [w9781 _]
                  frame Disabled {
                    n3770 = Unbundle By Name(w9781) -> ("总电压过低"=w9780:dbl)
                    n3771 = call "输入分辨率计算-EV05.vi"("1字节?"=FALSE, "数值"=w9780, "分辨率"=0.1) -> ("低字节"=w9783:dbl, "高字节1"=w9782:dbl)  [unwired: 2 in, 5 out]
                  }
                  frame Enabled {
                    w9786 = 255 ("高字节1")
                  }
                }
                n3772 = Build Array(w9778, w9779) -> (w9777:i32[])
              }
              frame 2 {
                # "温度过高"
                n3773 = disable-structure shown="启用" {
                  disable-tunnel: [w9793 255 ("高字节1")] -> w9789
                  disable-tunnel: w9787 -> [w9791 _]
                  frame Disabled {
                    n3774 = Unbundle By Name(w9791) -> ("温度过高"=w9790:dbl)
                    n3775 = call "输入分辨率计算-EV05.vi"("1字节?"=TRUE, "数值"=w9790, "偏移量"=-40.0, "分辨率"=1.0) -> ("高字节1"=w9793:dbl)  [unwired: 1 in, 6 out]
                  }
                  frame Enabled {
                  }
                }
                n3776 = Build Array(w9789) -> (w9788:i32[])
              }
              frame 3 {
                # "温度过低"
                n3777 = disable-structure shown="启用" {
                  disable-tunnel: [w9803 255 ("高字节1")] -> w9799
                  disable-tunnel: w9797 -> [w9801 _]
                  frame Disabled {
                    n3778 = Unbundle By Name(w9801) -> ("温度过低"=w9800:dbl)
                    n3779 = call "输入分辨率计算-EV05.vi"("1字节?"=TRUE, "数值"=w9800, "偏移量"=-40.0, "分辨率"=1.0) -> ("高字节1"=w9803:dbl)  [unwired: 1 in, 6 out]
                  }
                  frame Enabled {
                  }
                }
                n3780 = Build Array(w9799) -> (w9798:i32[])
              }
              frame 4 {
                # "整组温度不均衡"
                n3781 = disable-structure shown="启用" {
                  disable-tunnel: [w9813 255 ("高字节1")] -> w9809
                  disable-tunnel: w9807 -> [w9811 _]
                  frame Disabled {
                    n3782 = Unbundle By Name(w9811) -> ("整组温度不均衡"=w9810:dbl)
                    n3783 = call "输入分辨率计算-EV05.vi"("1字节?"=TRUE, "数值"=w9810, "偏移量"=0.0, "分辨率"=1.0) -> ("高字节1"=w9813:dbl)  [unwired: 1 in, 6 out]
                  }
                  frame Enabled {
                  }
                }
                n3784 = Build Array(w9809) -> (w9808:i32[])
              }
              frame 5 {
                # "单组电压不均衡"
                n3785 = disable-structure shown="启用" {
                  disable-tunnel: [w9825 w9828] -> w9820
                  disable-tunnel: [w9823 w9828] -> w9818
                  disable-tunnel: w9817 -> [w9822 _]
                  frame Disabled {
                    n3786 = Unbundle By Name(w9822) -> ("单组电压不均衡"=w9821:dbl)
                    n3787 = call "输入分辨率计算-EV05.vi"("1字节?"=FALSE, "数值"=w9821, "偏移量"=0.0, "分辨率"=0.001) -> ("低字节"=w9823:dbl, "高字节1"=w9825:dbl)  [unwired: 1 in, 5 out]
                  }
                  frame Enabled {
                    w9828 = 255 ("高字节1")
                  }
                }
                n3788 = Build Array(w9820, w9818) -> (w9819:i32[])
              }
              frame 6 {
                # "整组电压不均衡"
                n3789 = disable-structure shown="启用" {
                  disable-tunnel: [w9837 w9840] -> w9832
                  disable-tunnel: [w9835 w9840] -> w9830
                  disable-tunnel: w9829 -> [w9834 _]
                  frame Disabled {
                    n3790 = Unbundle By Name(w9834) -> ("整组电压不均衡"=w9833:dbl)
                    n3791 = call "输入分辨率计算-EV05.vi"("1字节?"=FALSE, "数值"=w9833, "偏移量"=0.0, "分辨率"=0.001) -> ("低字节"=w9835:dbl, "高字节1"=w9837:dbl)  [unwired: 1 in, 5 out]
                  }
                  frame Enabled {
                    w9840 = 255 ("高字节1")
                  }
                }
                n3792 = Build Array(w9832, w9830) -> (w9831:i32[])
              }
              frame 7 {
                # "单体电压过高"
                n3793 = disable-structure shown="启用" {
                  disable-tunnel: [w9849 w9852] -> w9844
                  disable-tunnel: [w9847 w9852] -> w9842
                  disable-tunnel: w9841 -> [w9846 _]
                  frame Disabled {
                    n3794 = Unbundle By Name(w9846) -> ("单体电压过高"=w9845:dbl)
                    n3795 = call "输入分辨率计算-EV05.vi"("1字节?"=FALSE, "数值"=w9845, "偏移量"=0.0, "分辨率"=0.001) -> ("低字节"=w9847:dbl, "高字节1"=w9849:dbl)  [unwired: 1 in, 5 out]
                  }
                  frame Enabled {
                    w9852 = 255 ("高字节1")
                  }
                }
                n3796 = Build Array(w9844, w9842) -> (w9843:i32[])
              }
              frame 8 {
                # "单体电压过低"
                n3797 = disable-structure shown="启用" {
                  disable-tunnel: [w9861 w9864] -> w9856
                  disable-tunnel: [w9859 w9864] -> w9854
                  disable-tunnel: w9853 -> [w9858 _]
                  frame Disabled {
                    n3798 = Unbundle By Name(w9858) -> ("单体电压过低"=w9857:dbl)
                    n3799 = call "输入分辨率计算-EV05.vi"("1字节?"=FALSE, "数值"=w9857, "偏移量"=0.0, "分辨率"=0.001) -> ("低字节"=w9859:dbl, "高字节1"=w9861:dbl)  [unwired: 1 in, 5 out]
                  }
                  frame Enabled {
                    w9864 = 255 ("高字节1")
                  }
                }
                n3800 = Build Array(w9856, w9854) -> (w9855:i32[])
              }
              frame 9 {
                # "充电电流过高"
                n3801 = disable-structure shown="启用" {
                  disable-tunnel: [w9873 w9876] -> w9868
                  disable-tunnel: [w9871 w9876] -> w9866
                  disable-tunnel: w9865 -> [w9870 _]
                  frame Disabled {
                    n3802 = Unbundle By Name(w9870) -> ("充电电流过高"=w9869:dbl)
                    n3803 = call "输入分辨率计算-EV05.vi"("1字节?"=FALSE, "数值"=w9869, "偏移量"=-3000.0, "分辨率"=0.1) -> ("低字节"=w9871:dbl, "高字节1"=w9873:dbl)  [unwired: 1 in, 5 out]
                  }
                  frame Enabled {
                    w9876 = 255 ("高字节1")
                  }
                }
                n3804 = Build Array(w9868, w9866) -> (w9867:i32[])
              }
              frame 10 {
                # "放电电流过高"
                n3805 = disable-structure shown="启用" {
                  disable-tunnel: [w9885 w9888] -> w9880
                  disable-tunnel: [w9883 w9888] -> w9878
                  disable-tunnel: w9877 -> [w9882 _]
                  frame Disabled {
                    n3806 = Unbundle By Name(w9882) -> ("放电电流过高"=w9881:dbl)
                    n3807 = call "输入分辨率计算-EV05.vi"("1字节?"=FALSE, "数值"=w9881, "偏移量"=-3000.0, "分辨率"=0.1) -> ("低字节"=w9883:dbl, "高字节1"=w9885:dbl)  [unwired: 1 in, 5 out]
                  }
                  frame Enabled {
                    w9888 = 255 ("高字节1")
                  }
                }
                n3808 = Build Array(w9880, w9878) -> (w9879:i32[])
              }
              frame 11 {
                # "单组温度不均衡"
                n3809 = disable-structure shown="启用" {
                  disable-tunnel: [w9895 255 ("高字节1")] -> w9891
                  disable-tunnel: w9889 -> [w9893 _]
                  frame Disabled {
                    n3810 = Unbundle By Name(w9893) -> ("单组温度不均衡"=w9892:dbl)
                    n3811 = call "输入分辨率计算-EV05.vi"("1字节?"=TRUE, "数值"=w9892, "偏移量"=0.0, "分辨率"=1.0) -> ("高字节1"=w9895:dbl)  [unwired: 1 in, 6 out]
                  }
                  frame Enabled {
                  }
                }
                n3812 = Build Array(w9891) -> (w9890:i32[])
              }
              frame 12 {
                # "SOC过高"
                n3813 = Unbundle By Name(w9903) -> ("SOC过高"=w9902:dbl)
                n3814 = call "输入分辨率计算-EV05.vi"("1字节?"=FALSE, "数值"=w9902, "偏移量"=0.0, "分辨率"=0.1) -> ("低字节"=w9904:dbl, "高字节1"=w9905:dbl)  [unwired: 1 in, 5 out]
                n3815 = call "二进制解析-8.6.vi"("索引"=4, "数值"=w9905) -> ("低位子数组"=w9908:i32[])  [unwired: 3 out]
                n3816 = call "二进制解析-8.6.vi"("索引"=4, "数值"=w9904) -> ("低位子数组"=w9900:i32[], "高位子数组"=w9907:i32[])  [unwired: 2 out]
                n3817 = Insert Into Array(array=w9908, new element=w9907) -> (w9906:i32[])  [unwired: 1 in]
                n3818 = call "数值二进制转十进制-8.6.vi"("子数组"=w9906) -> ("十进制数值"=w9901:i32)  [unwired: 4 out]
                n3819 = disable-structure shown="启用" {
                  disable-tunnel: w9901 -> [w9916 _]
                  disable-tunnel: [w9916 255 ("高字节1")] -> w9899
                  disable-tunnel: w9900 -> [w9915 _]
                  disable-tunnel: [w9915 i32[] [] ("低位子数组 29")] -> _
                  frame Disabled {
                  }
                  frame Enabled {
                  }
                }
                n3820 = Build Array(w9899, w9899) -> (w9912:i32[])
              }
              frame 13 {
                # "SOC过低"
                n3821 = Unbundle By Name(w9924) -> ("SOC过低"=w9923:dbl)
                n3822 = call "输入分辨率计算-EV05.vi"("1字节?"=FALSE, "数值"=w9923, "偏移量"=0.0, "分辨率"=0.1) -> ("低字节"=w9921:dbl, "高字节1"=w9922:dbl)  [unwired: 1 in, 5 out]
                n3823 = call "二进制解析-8.6.vi"("索引"=4, "数值"=w9922) -> ("低位子数组"=w9920:i32[])  [unwired: 3 out]
                n3824 = disable-structure shown="启用" {
                  disable-tunnel: w9921 -> [w9931 _]
                  disable-tunnel: [w9931 255 ("高字节1")] -> w9919
                  disable-tunnel: w9920 -> [w9930 _]
                  disable-tunnel: [w9930 i32[] [] ("低位子数组")] -> _
                  frame Disabled {
                    (unwired) i32[] [] ("低位子数组 4")
                  }
                  frame Enabled {
                  }
                }
                n3825 = Build Array(w9919, w9919) -> (w9927:i32[])
              }
              frame 14 {
                # "内阻过大"
                n3826 = disable-structure shown="启用" {
                  disable-tunnel: w9936 -> [w9941 _]
                  disable-tunnel: [w9937 255 ("高字节1")] -> w9934
                  frame Enabled {
                    n3827 = Unbundle By Name(w9941) -> ("内阻过大"=w9940:dbl)
                    n3828 = call "输入分辨率计算-EV05.vi"("1字节?"=TRUE, "数值"=w9940, "分辨率"=0.1) -> ("高字节1"=w9937:dbl)  [unwired: 2 in, 6 out]
                  }
                  frame Disabled {
                  }
                }
